vi "Point by point acquistion.vi"() -> ()   [LabVIEW 2010]
panel:
  out "Error Code":i32
  out "Error Message":string
  in  "Channel":i32=1
  in  "BoardNum":u32
  out "Waveform Chart":u16(graph)
  in  "STOP":bool
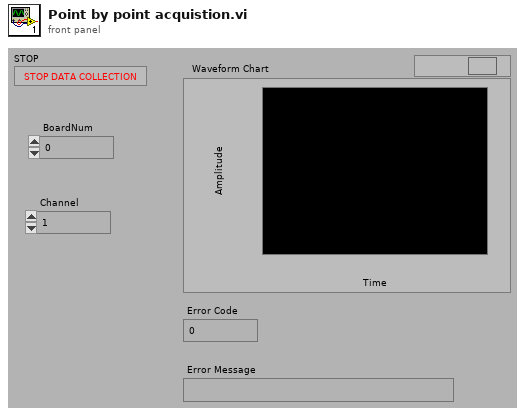
[diagram p1: front panel]
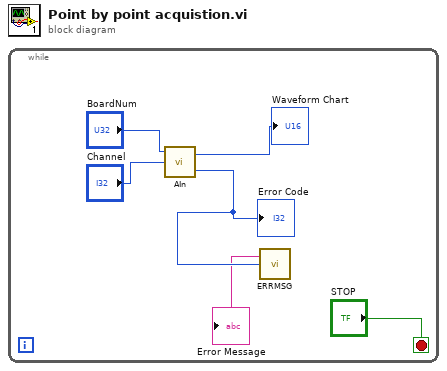
[diagram p0: block diagram]
diagram:
  n1 = while {
    stop <- "STOP" stop-if-true
    n2 = call <menus>:"AIn.VI"("Channel"="Channel", "BoardNum"="BoardNum") -> ("ErrCode"=w2:i32, "DataValue"=→"Waveform Chart":u16)  [unwired: 1 in]
    "Error Code" <- w2
    n3 = call <menus>:"ERRMSG.VI"("ErrCode"=w2) -> ("ErrMsg"=→"Error Message":string)  [unwired: 1 out]
  }
